vi "File to Number Array.vi"(8 "error in":errorcluster, 11 "file path":path) -> (0 "error out":errorcluster, 2 "text":string, 3 "Array":i32[](array[numeric]))   [LabVIEW 2014]
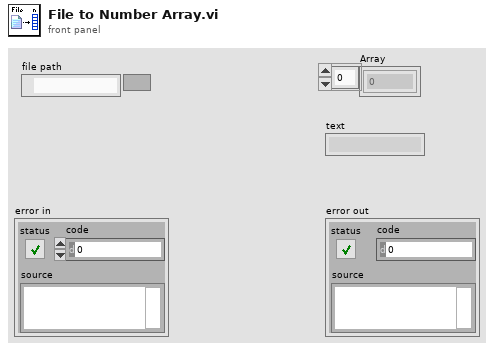
[diagram p1: front panel]
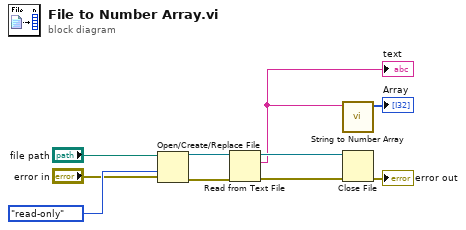
[diagram p0: block diagram]
diagram:
  n1 = Open/Create/Replace File(file path (use dialog)="file path", error in="error in", access (0:read/write)=enum16{"read/write", "read-only", "write-only"}."read-only") -> (refnum out=w10:refnum<file>, error out=w8:errorcluster)  [unwired: 3 in, 1 out]
  n2 = Read from Text File(file (use dialog)=w10, error in=w8) -> (refnum out=w9:refnum<file>, text=w4:string, error out=w7:errorcluster)  [unwired: 2 in, 1 out]
  "text" <- w4
  n3 = call "String to Number Array.vi"("Input String"=w4) -> ("Array"=→"Array":i32[])  [unwired: 10 in]
  n4 = Close File(refnum=w9, error in=w7) -> (error out=→"error out":errorcluster)  [unwired: 1 out]
